vi "DataTypeExperiments.vi"() -> ()   [LabVIEW 2018]
panel:
  out "B 2":dbl
  out "G 2":dbl
  out "R 2":dbl
  out "index (row)":i32
  out "Array 4":u32[][](array[colorbox])
  in  "Index":i32
  out "String":string
  out "Array 3":dbl[](array[slide]) scale=0.0..10.0
  out "size(s)":i32
  in  "Array 2":i32[](array[numeric])
  out "Array":i32[](array[slide]) scale=0.0..10.0
  out "B":dbl
  out "G":dbl
  out "R":dbl
  out "Color":u32(colorbox)
  in  "stop":bool
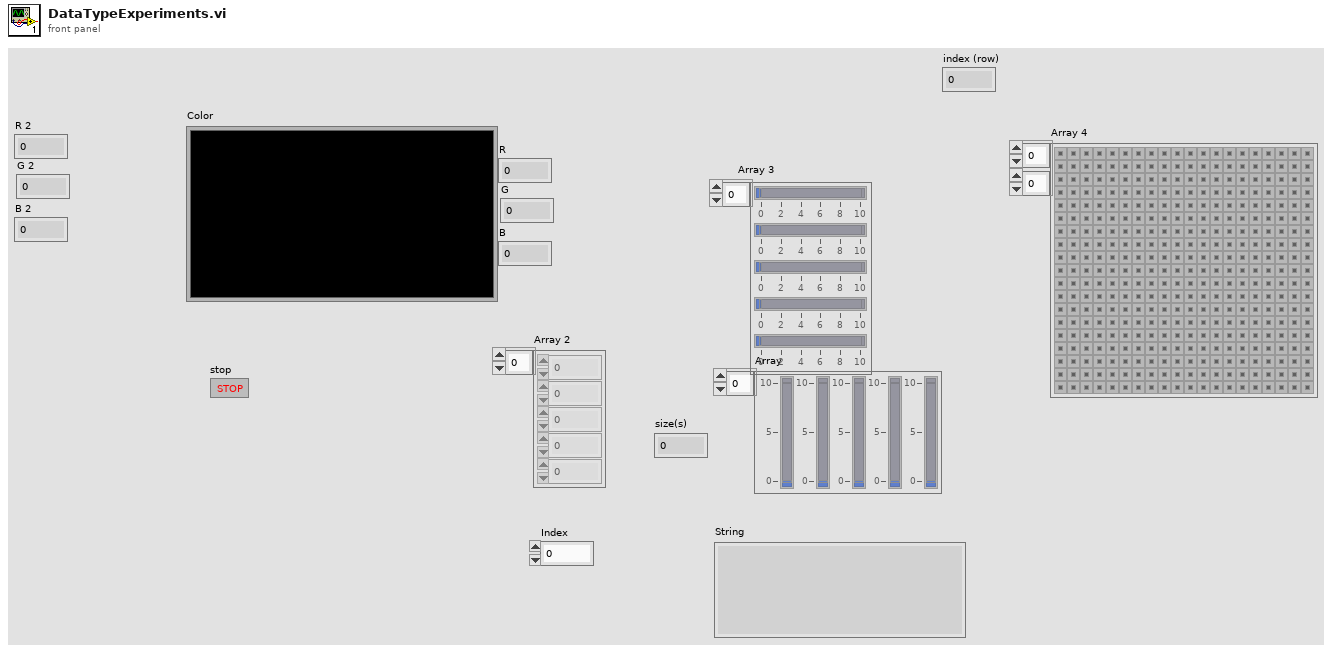
[diagram p1: front panel]
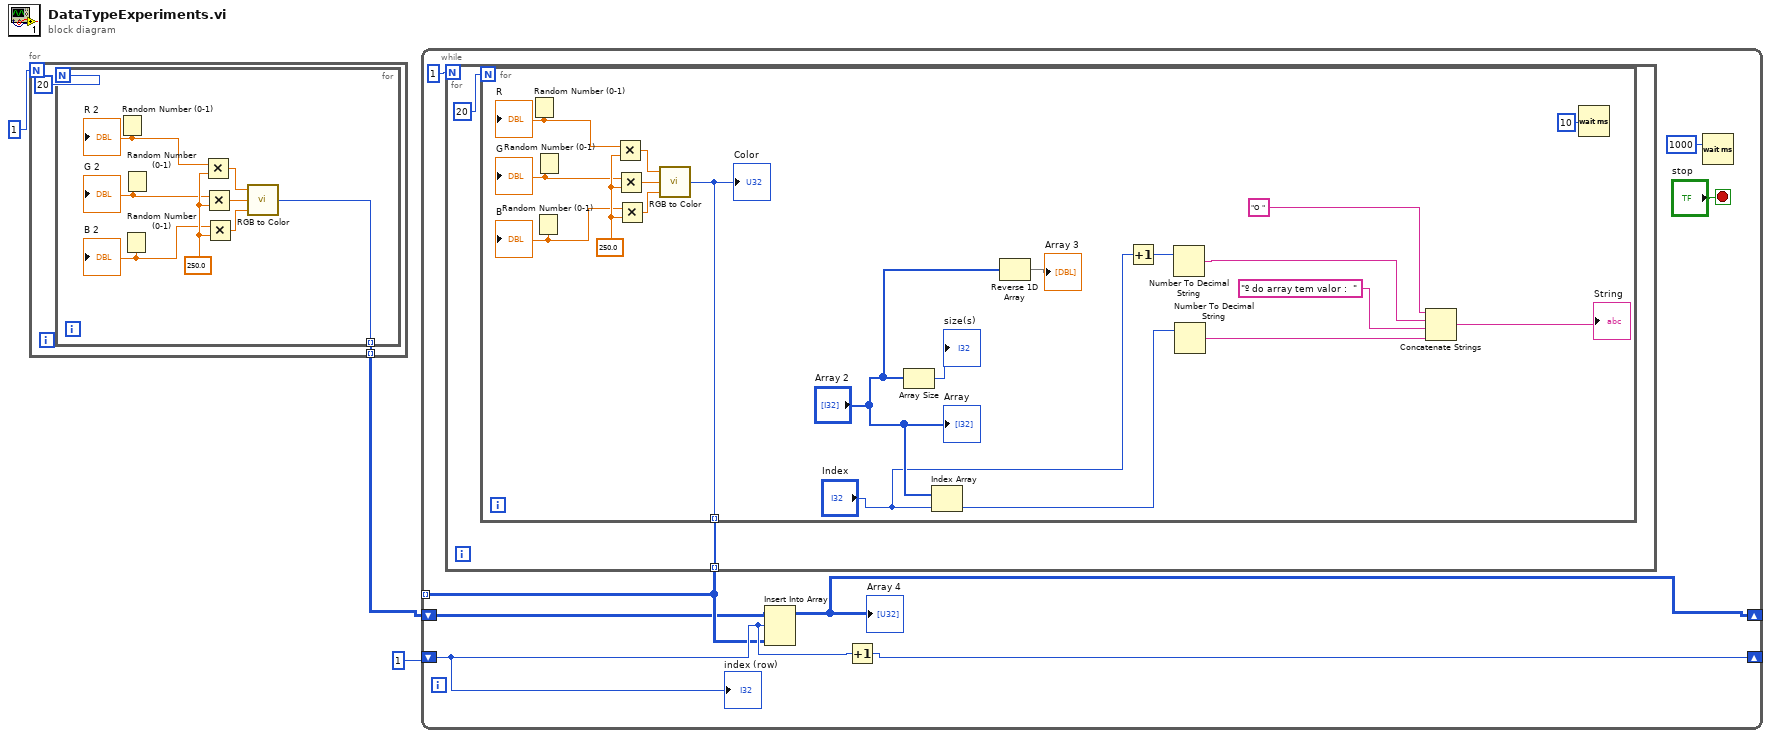
[diagram p0: block diagram]
diagram:
  n1 = for {
    N: 1 -> [_]
    tunnel: [w4] -> w1 mode=indexing
    n2 = for {
      N: 20 -> [_]
      tunnel: [w6] -> w4 mode=indexing
      w13 = 250.0
      n3 = Random Number (0-1)() -> (number: 0 to 1=w7:dbl)
      "R 2" <- w7
      n4 = Random Number (0-1)() -> (number: 0 to 1=w9:dbl)
      "B 2" <- w9
      n5 = Random Number (0-1)() -> (number: 0 to 1=w8:dbl)
      "G 2" <- w8
      n6 = Multiply(x=w7, y=w13) -> (x*y=w10:dbl)
      n7 = Multiply(x=w8, y=w13) -> (x*y=w11:dbl)
      n8 = Multiply(x=w9, y=w13) -> (x*y=w12:dbl)
      n9 = call <vilib>:"RGB to Color.vi"("B"=w12, "G"=w11, "R"=w10) -> ("Color"=w6:u32)
    }
  }
  n10 = while {
    shift-right: [w14] -> _
    shift-left: w1 -> [w15]
    shift-right: [w18] -> _
    shift-left: 1 ("index (row)") -> [w17]
    tunnel: [w16] -> _ mode=indexing
    stop <- "stop" stop-if-true
    n11 = for {
      N: 1 -> [_]
      tunnel: [w22] -> w16 mode=indexing
      n12 = for {
        N: 20 -> [_]
        tunnel: [w25] -> w22 mode=indexing
        w43 = 250.0
        n13 = Random Number (0-1)() -> (number: 0 to 1=w37:dbl)
        "R" <- w37
        n14 = Random Number (0-1)() -> (number: 0 to 1=w39:dbl)
        "B" <- w39
        n15 = Random Number (0-1)() -> (number: 0 to 1=w38:dbl)
        "G" <- w38
        n16 = Multiply(x=w37, y=w43) -> (x*y=w40:dbl)
        n17 = Multiply(x=w38, y=w43) -> (x*y=w41:dbl)
        n18 = Multiply(x=w39, y=w43) -> (x*y=w42:dbl)
        n19 = call <vilib>:"RGB to Color.vi"("B"=w42, "G"=w41, "R"=w40) -> ("Color"=w25:u32)
        "Color" <- w25
        n20 = Array Size(array="Array 2") -> (size(s)=→"size(s)":i32)
        n21 = Index Array(array="Array 2", index="Index") -> (element=w30:i32)
        n22 = Reverse 1D Array(array="Array 2") -> (reversed array=→"Array 3":i32[])
        n23 = Increment(x="Index") -> (x+1=w26:i32)
        n24 = Number To Decimal String(number=w26) -> (decimal integer string=w32:string)  [unwired: 1 in]
        n25 = Number To Decimal String(number=w30) -> (decimal integer string=w29:string)  [unwired: 1 in]
        n26 = Concatenate Strings("O ", w32, "º do array tem valor :  ", w29) -> (→"String":string)
        n27 = Wait (ms)(milliseconds to wait=u32 10) -> ()  [unwired: 1 out]
        "Array" <- "Array 2"
      }
    }
    n28 = Insert Into Array(array=w15, index (row)=w17, new element=w16) -> (w14:u32[][])  [unwired: 1 in]
    "Array 4" <- w14
    n29 = Increment(x=w17) -> (x+1=w18:i32)
    n30 = Wait (ms)(milliseconds to wait=u32 1000) -> ()  [unwired: 1 out]
    "index (row)" <- w17
  }
